vi "Write value.vi"(8 "error in (no error)":errorcluster, 10 "value":variant, 11 "JSON Value in":refnum<class "JSON Value.lvclass">) -> (0 "error out":errorcluster, 3 "JSON Value out":refnum<class "JSON Value.lvclass">)   [LabVIEW 2016, in "JSON Value.lvclass"]
uses:
  JSON Value.lvclass
  JSON Value.lvclass/JSON Value.ctl
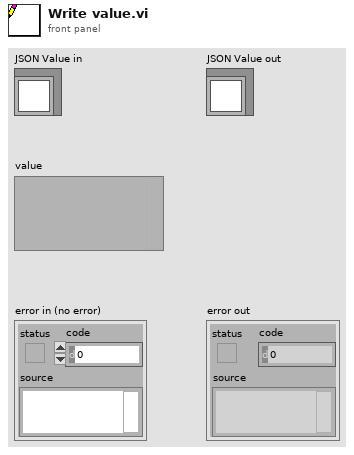
[diagram p1: front panel]
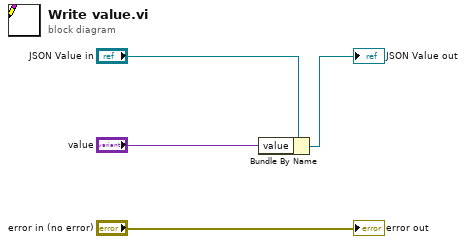
[diagram p0: block diagram]
diagram:
  n1 = Bundle By Name(cluster="JSON Value in", "value"="value") -> (→"JSON Value out":refnum<class "JSON Value.lvclass">)
  "error out" <- "error in (no error)"
